vi "持续运行的加法.vi"() -> ()   [LabVIEW 2021]
doc: "本VI是为《我和LabVIEW》一书编写的示例。\n关于本书的介绍请参考网页：\nhttp://ruanqizhen.spaces.live.com/blog/cns!5852D4F797C53FB6!4310.entry"
panel:
  in  "停止":bool
  out "量表":dbl(knob) scale=0.0..20.0
  in  "è½¬ç›˜ÅÌ":dbl(knob) scale=0.0..10.0
  in  "旋钮":dbl(knob) scale=0.0..10.0
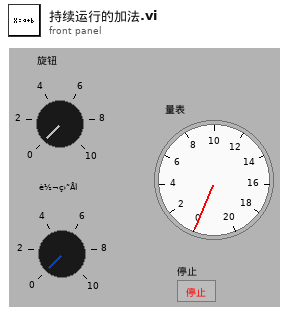
[diagram p1: front panel]
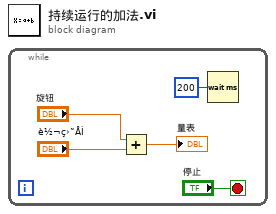
[diagram p0: block diagram]
diagram:
  n1 = while {
    stop <- "停止" stop-if-true
    n2 = Add(x="旋钮", y="è½¬ç›˜ÅÌ") -> (x+y=→"量表":dbl)
    n3 = Wait (ms)(milliseconds to wait=u32 200 ("等待时间（毫秒）")) -> ()  [unwired: 1 out]
  }
